vi "StartCore.vi"(8 "error in (no error)":errorcluster, 9 "Simulate?":bool, 10 "Service Details In":T1, 11 "MicronGRPCClient in":refnum<class "MicronGRPCClient.lvclass">) -> (0 "error out":errorcluster, 1 "Service Details Out":T1, 2 "Connection String":string, 3 "MicronGRPCClient out":refnum<class "MicronGRPCClient.lvclass">)   [LabVIEW 2019, in "MicronGRPCClient.lvclass"]
uses:
  MicronGRPCClient.lvclass
  Base/Client/Typedefs/ServiceDetails.ctl
  d0e40df4-b580-449e-8344-b3b1466a123c.vi
  MicronCLI/MicronCLI.lvclass
  Base/Client/MicronClient.lvclass
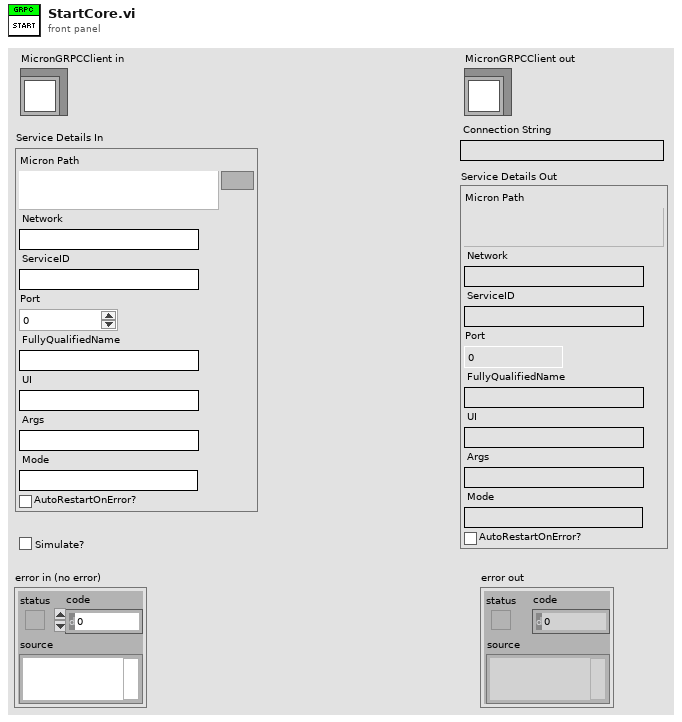
[diagram p1: front panel]
types:
  T1 = typedef "MicronClient.lvclass/ServiceDetails.ctl" = cluster{"Micron Path":path, "Network":string, "ServiceID":string, "Port":i32, "FullyQualifiedName":string, "UI":string, "Args":string, "Mode":string, "AutoRestartOnError?":bool}
  T2 = typedef "MicronCLI.lvclass/ServiceDetails.ctl" = cluster{"Network":string, "ServiceID":string}
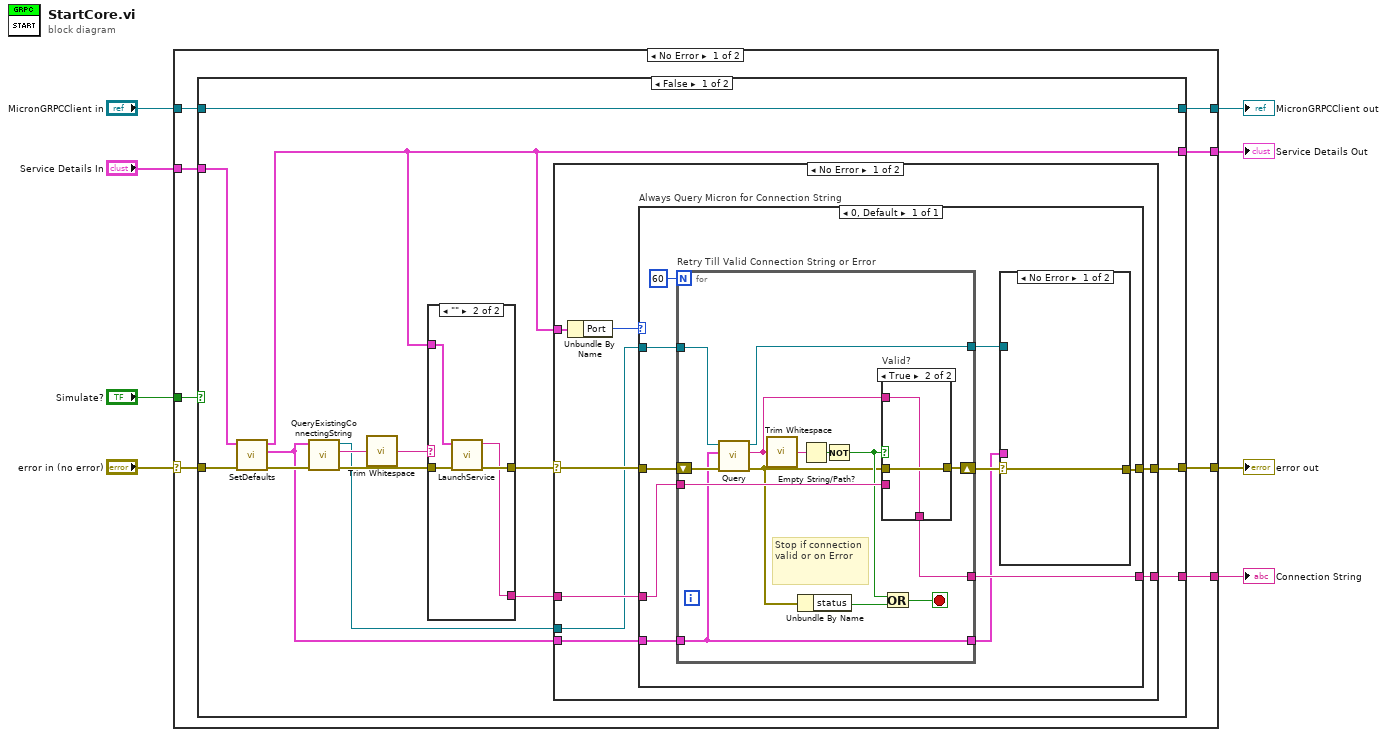
[diagram p0: block diagram]
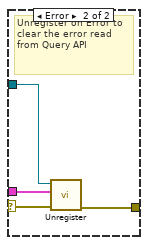
[diagram p2: hidden frame]
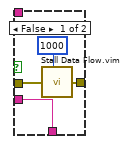
[diagram p3: hidden frame]
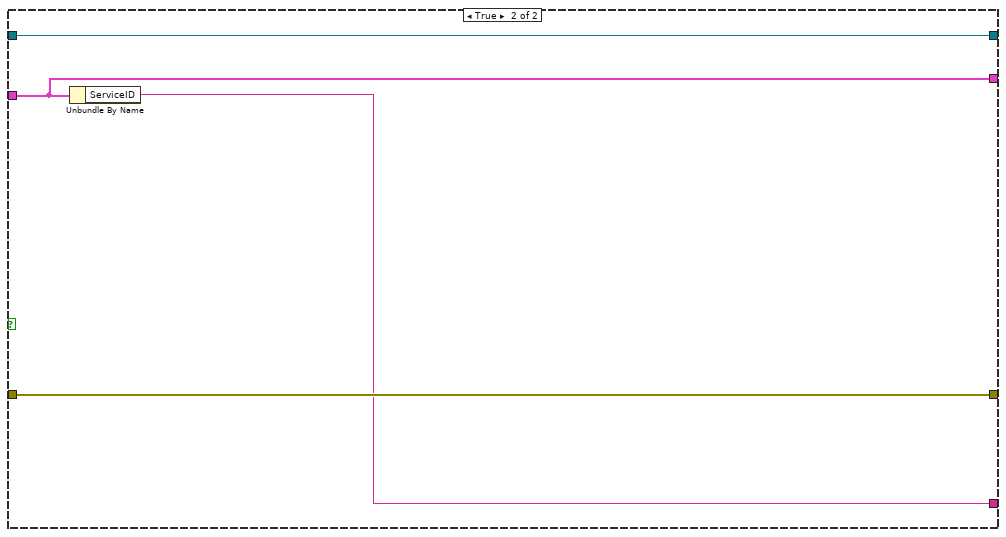
[diagram p6: hidden frame]
diagram:
  n1 = case shown="No Error" "error in (no error)" {
    selector: "error in (no error)" -> [w14 w88]
    tunnel: [w16 w88] -> w8
    tunnel: [w11 w87] -> w5
    tunnel: "MicronGRPCClient in" -> [w10 w87]
    tunnel: [w13 _] -> w6
    tunnel: "Service Details In" -> [w15 w86]
    tunnel: "Simulate?" -> [w12 _]
    tunnel: [w9 w86] -> w7
    frame No Error {
      n2 = case shown="False" w12 {
        tunnel: [w24 w85] -> w16
        tunnel: w15 -> [w30 w82]
        tunnel: w14 -> [w29 w85]
        tunnel: [w25 w83] -> w13
        tunnel: [w17 w84] -> w11
        tunnel: w10 -> [w17 w84]
        tunnel: [w18 w82] -> w9
        frame False {
          n3 = call "SetDefaults.vi"("error in (no error)"=w29, "Service Details In"=w30) -> ("error out"=w28:errorcluster, "Service"=w20:T2, "Service Details Out"=w18:T1)  [unwired: 7 in]
          n4 = call "QueryExistingConnectingString.vi"("error in (no error)"=w28, "Service"=w20) -> ("error out"=w23:errorcluster, "Connection String"=w22:string, "MicronCLI out"=w21:refnum<class "MicronCLI.lvclass">)  [unwired: 7 in]
          n5 = call <vilib>:"Trim Whitespace.vi"("string"=w22) -> ("trimmed string"=w19:string)  [unwired: 1 in]
          n6 = case shown="\"\"" w19 {
            selector: w19 -> [w77 _]
            tunnel: [w76 w81] -> w26
            tunnel: w18 -> [_ w78]
            tunnel: [w77 w80] -> w27
            tunnel: w23 -> [w76 w79]
            frame Default {
            }
            frame "" {
              n7 = call "LaunchService.vi"("error in (no error)"=w79, "Service Details Out"=w78) -> ("error out"=w81:errorcluster, "Default Connection String"=w80:string)  [unwired: 8 in]
            }
          }
          n8 = case shown="No Error" w26 {
            selector: w26 -> [w35 w75]
            tunnel: w27 -> [w38 w74]
            tunnel: w18 -> [w37 _]
            tunnel: [w34 w74] -> w25
            tunnel: [w33 w75] -> w24
            tunnel: w21 -> [w32 _]
            tunnel: w20 -> [w31 _]
            frame No Error {
              n9 = Unbundle By Name(w37) -> ("Port"=w36:i32)
              n10 = case "Always Query Micron for Connection String" shown="0, Default" w36 {
                tunnel: w38 -> [w44]
                tunnel: w35 -> [w48]
                tunnel: [w45] -> w34
                tunnel: [w41] -> w33
                tunnel: w32 -> [w47]
                tunnel: w31 -> [w43]
                frame 0, Default {
                  n11 = for "Retry Till Valid Connection String or Error" {
                    N: 60 -> [_]
                    tunnel: w47 -> [w56]
                    shift-right: [w66] -> w42
                    shift-left: w48 -> [w67]
                    tunnel: [w65] -> w45
                    tunnel: w44 -> [w64]
                    tunnel: w43 -> [w55]
                    tunnel: [w54] -> w40
                    tunnel: [w55] -> w39
                    stop <- w58 stop-if-true
                    # "Stop if connection valid or on Error"
                    n12 = call-dynamic "Query.vi"("error in (no error)"=w67, "Service"=w55, "MicronCLI in"=w56) -> ("error out"=w59:errorcluster, "ConnectionString"=w62:string, "MicronCLI out"=w54:refnum<class "MicronCLI.lvclass">)  [unwired: 6 in]
                    n13 = call <vilib>:"Trim Whitespace.vi"("string"=w62) -> ("trimmed string"=w63:string)  [unwired: 1 in]
                    n14 = Unbundle By Name(w59) -> ("status"=w57:bool)
                    n15 = Empty String/Path?(string/path=w63) -> (empty?=w61:bool)
                    n16 = Not(x=w61) -> (.not. x?=w60:bool)
                    n17 = case "Valid?" shown="True" w60 {
                      tunnel: w59 -> [w71 w73]
                      tunnel: [w70 w73] -> w66
                      tunnel: [w69 w72] -> w65
                      tunnel: w64 -> [w69 _]
                      tunnel: w62 -> [_ w72]
                      frame False {
                        n18 = call "Stall Data Flow.vim"("value in"=w71, "milliseconds to wait"=u32 1000) -> ("value out"=w70:errorcluster)  [unwired: 1 out]
                      }
                      frame True {
                      }
                    }
                    n19 = Or(x=w60, y=w57) -> (x .or. y?=w58:bool)
                  }
                  n20 = case shown="No Error" w42 {
                    selector: w42 -> [w49 w53]
                    tunnel: [w49 w52] -> w41
                    tunnel: w40 -> [_ w51]
                    tunnel: w39 -> [_ w50]
                    frame No Error {
                    }
                    frame Error {
                      # "Unregister on Error to clear the error read from Query API"
                      n21 = call-dynamic "Unregister.vi"("error in (no error)"=w53, "Service"=w50, "MicronCLI in"=w51) -> ("error out"=w52:errorcluster)  [unwired: 7 in, 1 out]
                    }
                  }
                }
              }
            }
            frame Error {
            }
          }
        }
        frame True {
          n22 = Unbundle By Name(w82) -> ("ServiceID"=w83:string)
        }
      }
    }
    frame Error {
    }
  }
  "error out" <- w8
  "MicronGRPCClient out" <- w5
  "Connection String" <- w6
  "Service Details Out" <- w7
